vi "Method.vi"(4 "Value":refnum<class "Abs_Numeric.lvclass">) -> (1 "Result":refnum<class "ConvertTo_CPLX_EXT.lvclass">)   [LabVIEW 2021, in "ConvertTo_CPLX_EXT.lvclass"]
uses:
  ConvertTo_CPLX_EXT.lvclass
  Abs_Types/Numeric/Abs_Numeric.lvclass
  ConvertTo_CPLX_EXT.lvclass/ConvertTo_CPLX_EXT.ctl
  Properties/Write Value.vi
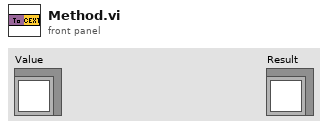
[diagram p1: front panel]
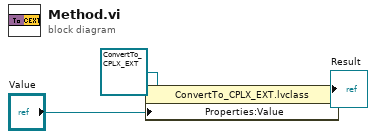
[diagram p0: block diagram]
diagram:
  n1 = property class="ConvertTo_CPLX_EXT.lvclass"(reference=refnum<class "ConvertTo_CPLX_EXT.lvclass"> refnum ("ConvertTo_DBL.lvclass"), "Properties:Value"="Value") -> (reference out=→"Result":refnum<class "ConvertTo_CPLX_EXT.lvclass">)  [unwired: 1 in, 1 out]
